vi "Create Enum.vi"(8 "error in (no error)":errorcluster, 9 "Choices":string[](array[string]), 10 "BaseType":refnum<class "LVType.lvclass">, 11 "ID":string) -> (0 "error out":errorcluster, 3 "LVEnum out":refnum<class "LVEnum.lvclass">)   [LabVIEW 2020, in "LVDataTypes.lvlib" / "LVEnum.lvclass"]
uses:
  <vilib>/AppBuilder/Engine/WebServiceDescription/LVDataTypes/LVEnum/LVEnum.lvclass
  e:/builds/penguin/labview/branches/2020/dev/dist/vi.lib/AppBuilder/Engine/WebServiceDescription/LVDataTypes/LVType/LVType.lvclass
  <vilib>/AppBuilder/Engine/WebServiceDescription/LVDataTypes/LVType/LVType.lvclass
  <vilib>/AppBuilder/Engine/WebServiceDescription/LVDataTypes/TypeCode.ctl
  <vilib>/AppBuilder/Engine/WebServiceDescription/LVDataTypes/LVEnum/LVEnum.lvclass/LVEnum.ctl
  <vilib>/AppBuilder/Engine/WebServiceDescription/LVDataTypes/LVDataTypes.lvlib
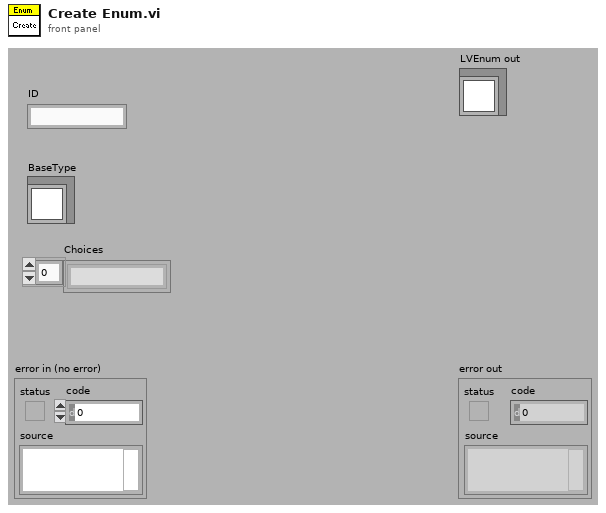
[diagram p1: front panel]
types:
  T1 = typedef "LVDataTypes.lvlib/TypeCode.ctl" = enum16{"Undefined", "Byte", "Unsigned Byte", "Word", "Unsigned Word", "Long", "Unsigned Long", "Quad", "Unsigned Quad", "Single", "Double", "Extended", "Enum", "Boolean", "String", "Path", "Array", "Cluster", "AnalogWaveform", "DigitalWaveform", "Time Stamp", "Void", "Complex Single", "Complex Double", "Complex Extended"}
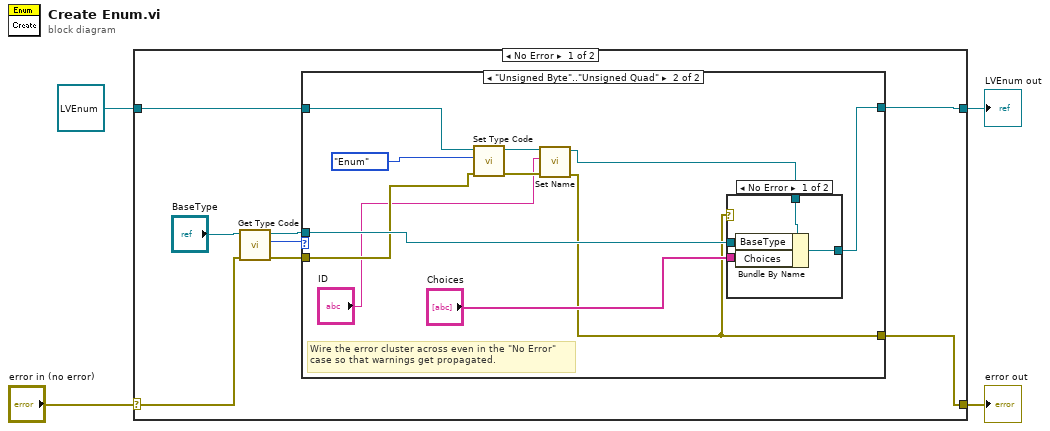
[diagram p0: block diagram]
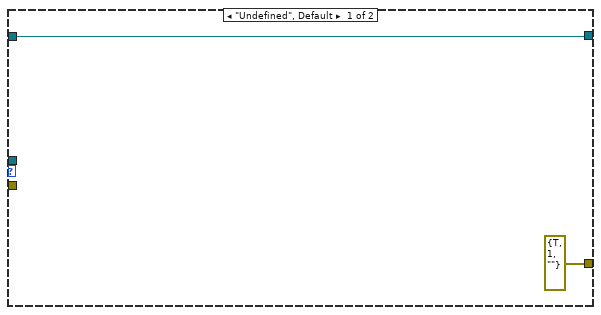
[diagram p2: hidden frame]
diagram:
  n1 = case shown="No Error" "error in (no error)" {
    selector: "error in (no error)" -> [w11 w32]
    tunnel: [w5 w32] -> w3
    tunnel: [w6 w31] -> w1
    tunnel: refnum<class "LVEnum.lvclass"> refnum ("LVEnum in") -> [w8 w31]
    frame No Error {
      n2 = call <vilib>:"Get Type Code.vi"("error in (no error)"=w11, "LVType.lvclass in"="BaseType") -> ("error out"=w9:errorcluster, "Type"=w10:T1, "LVType.lvclass out"=w7:refnum<class "LVType.lvclass">)  [unwired: 7 out]
      n3 = case shown="\"Unsigned Byte\"..\"Unsigned Quad\"" w10 {
        tunnel: w9 -> [_ w18]
        tunnel: w8 -> [w13 w20]
        tunnel: w7 -> [_ w25]
        tunnel: [w13 w23] -> w6
        tunnel: [errorcluster {"status"=TRUE, "code"=1, "source"=""} ("error out") w15] -> w5
        frame "Undefined", Default {
        }
        frame "Unsigned Byte".."Unsigned Quad" {
          # "Wire the error cluster across even in the \"No Error\"\ncase so that warnings get propagated."
          n4 = call <vilib>:"Set Type Code.vi"("error in (no error)"=w18, "Type"=TypeCode."Enum", "LVType.lvclass in"=w20) -> ("error out"=w21:errorcluster, "LVType.lvclass out"=w22:refnum<class "LVEnum.lvclass">)  [unwired: 7 out]
          n5 = call <vilib>:"Set Name.vi"("error in (no error)"=w21, "Name"="ID", "LVType.lvclass in"=w22) -> ("error out"=w15:errorcluster, "LVType.lvclass out"=w16:refnum<class "LVEnum.lvclass">)  [unwired: 7 out]
          n6 = case shown="No Error" w15 {
            tunnel: w16 -> [w29 w30]
            tunnel: w25 -> [w28 _]
            tunnel: "Choices" -> [w27 _]
            tunnel: [w26 w30] -> w23
            frame No Error {
              n7 = Bundle By Name(cluster=w29, "BaseType"=w28, "Choices"=w27) -> (w26:refnum<class "LVEnum.lvclass">)
            }
            frame Error {
            }
          }
        }
      }
    }
    frame Error {
    }
  }
  "error out" <- w3
  "LVEnum out" <- w1
